vi "Add Default Free.vi"(8 "error in (no error)":errorcluster, 10 "ToModBus":bool, 11 "Thermocouple in":refnum<class "Thermocouple.lvclass">) -> (0 "error out":errorcluster, 3 "Thermocouple out":refnum<class "Thermocouple.lvclass">)   [LabVIEW 2018, in "Measurement Channels.lvlib" / "Thermocouple.lvclass"]
uses:
  Thermocouple.lvclass
  Thermocouple.lvclass/Thermocouple.ctl
  Class Channel/Channel.lvclass
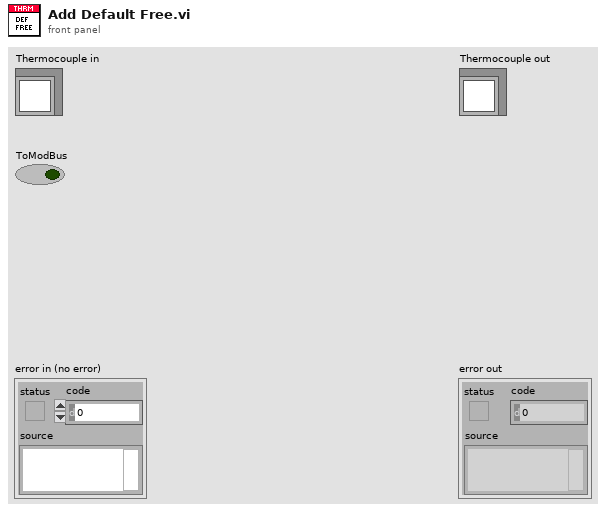
[diagram p1: front panel]
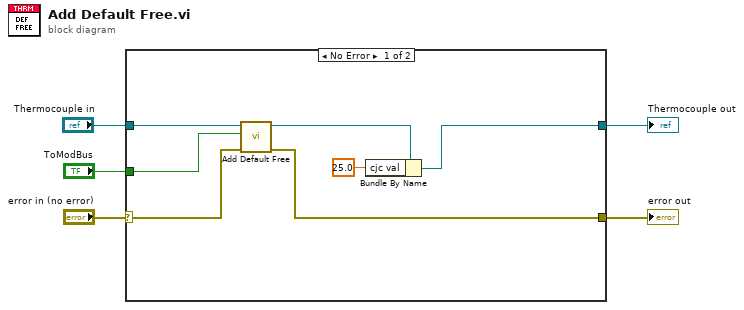
[diagram p0: block diagram]
diagram:
  n1 = case shown="No Error" "error in (no error)" {
    selector: "error in (no error)" -> [w9 w13]
    tunnel: [w12 w13] -> w5
    tunnel: [w6 w14] -> w4
    tunnel: "ToModBus" -> [w11 _]
    tunnel: "Thermocouple in" -> [w10 w14]
    frame No Error {
      n2 = call-parent "Add Default Free.vi"("error in (no error)"=w9, "ToModBus"=w11, "Channel in"=w10) -> ("error out"=w12:errorcluster, "Channel out"=w7:refnum<class "Thermocouple.lvclass">)  [unwired: 7 in]
      n3 = Bundle By Name(cluster=w7, "cjc val"=25.0 ("CJC Val")) -> (w6:refnum<class "Thermocouple.lvclass">)
    }
    frame Error {
    }
  }
  "error out" <- w5
  "Thermocouple out" <- w4
